vi "new8channelConvert.vi"(8 "Port 0":T1={"Port 0 Channel 0"=[0, 0, 0, 0, 0, 0, 0, 0, 0], "Port 0 Channel 1"=[0, 0, 0, 0, 0, 0, 0, 0, 0], "Port 0 Channel 2"=[0, 0, 0, 0, 0, 0, 0, 0, 0], "Port 0 Channel 3"=[0, 0, 0, 0, 0, 0, 0, 0, 0], "Port 0 Channel 4"=[0, 0, 0, 0, 0, 0, 0, 0, 0], "Port 0 Channel 5"=[0, 0, 0, 0, 0, 0, 0, 0, 0], "Port 0 Channel 6"=[0, 0, 0, 0, 0, 0, 0, 0, 0], "Port 0 Channel 7"=[0, 0, 0, 0, 0, 0, 0, 0, 0]}, 14 "采样率":i32=1, 18 "总时间（ms）":i32=10) -> (16 "单通道总采样点":i32, 19 "result":i32[](array[numeric]))   [LabVIEW 2021]
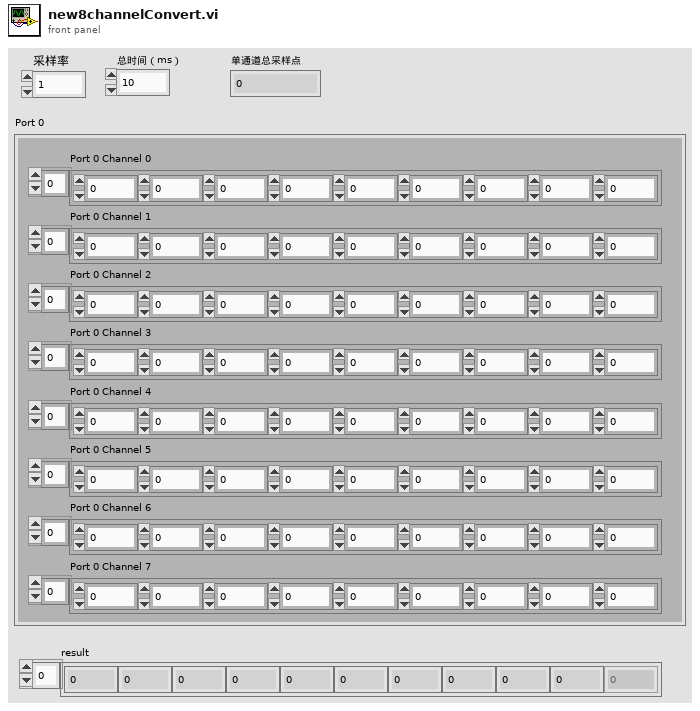
[diagram p1: front panel]
types:
  T1 = cluster{"Port 0 Channel 0":i32[], "Port 0 Channel 1":i32[], "Port 0 Channel 2":i32[], "Port 0 Channel 3":i32[], "Port 0 Channel 4":i32[], "Port 0 Channel 5":i32[], "Port 0 Channel 6":i32[], "Port 0 Channel 7":i32[]}
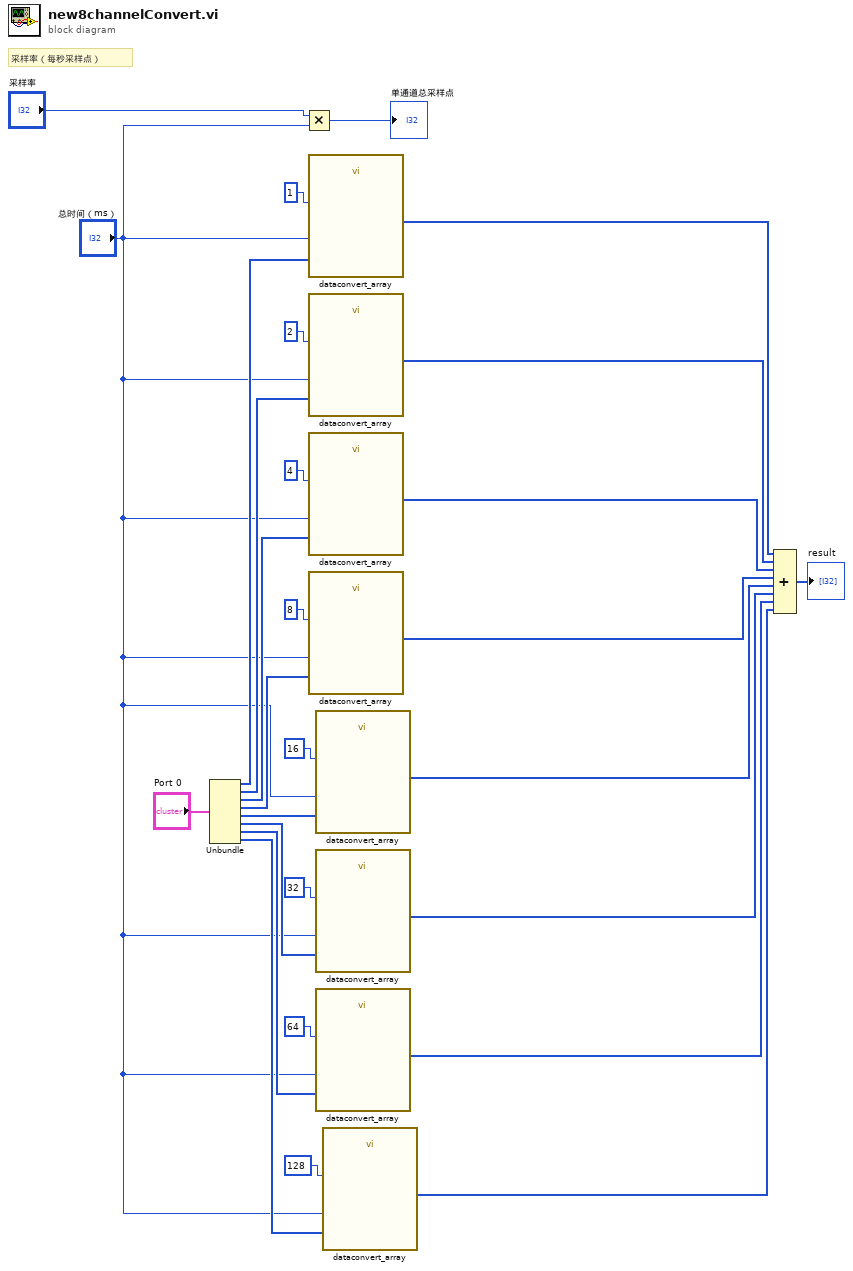
[diagram p0: block diagram]
diagram:
  # "采样率（每秒采样点）"
  n1 = Unbundle("Port 0") -> ("Port 0 Channel 0"=w20:i32[], "Port 0 Channel 1"=w19:i32[], "Port 0 Channel 2"=w18:i32[], "Port 0 Channel 3"=w17:i32[], "Port 0 Channel 4"=w16:i32[], "Port 0 Channel 5"=w15:i32[], "Port 0 Channel 6"=w14:i32[], "Port 0 Channel 7"=w13:i32[])
  n2 = Multiply(x="采样率", y="总时间（ms）") -> (x*y=→"单通道总采样点":i32)
  n3 = call "dataconvert_array.vi"("输入的TTL信号序列"=w20, "总时间（ms）"="总时间（ms）", "相乘倍数"=1) -> ("输出编码后的TTL序列"=w11:i32[])  [unwired: 8 in]
  n4 = call "dataconvert_array.vi"("输入的TTL信号序列"=w19, "总时间（ms）"="总时间（ms）", "相乘倍数"=2) -> ("输出编码后的TTL序列"=w10:i32[])  [unwired: 8 in]
  n5 = call "dataconvert_array.vi"("输入的TTL信号序列"=w18, "总时间（ms）"="总时间（ms）", "相乘倍数"=4) -> ("输出编码后的TTL序列"=w9:i32[])  [unwired: 8 in]
  n6 = call "dataconvert_array.vi"("输入的TTL信号序列"=w17, "总时间（ms）"="总时间（ms）", "相乘倍数"=8) -> ("输出编码后的TTL序列"=w8:i32[])  [unwired: 8 in]
  n7 = call "dataconvert_array.vi"("输入的TTL信号序列"=w16, "总时间（ms）"="总时间（ms）", "相乘倍数"=16) -> ("输出编码后的TTL序列"=w7:i32[])  [unwired: 8 in]
  n8 = call "dataconvert_array.vi"("输入的TTL信号序列"=w15, "总时间（ms）"="总时间（ms）", "相乘倍数"=32) -> ("输出编码后的TTL序列"=w6:i32[])  [unwired: 8 in]
  n9 = call "dataconvert_array.vi"("输入的TTL信号序列"=w14, "总时间（ms）"="总时间（ms）", "相乘倍数"=64) -> ("输出编码后的TTL序列"=w5:i32[])  [unwired: 8 in]
  n10 = call "dataconvert_array.vi"("输入的TTL信号序列"=w13, "总时间（ms）"="总时间（ms）", "相乘倍数"=128) -> ("输出编码后的TTL序列"=w4:i32[])  [unwired: 8 in]
  n11 = Compound Arithmetic op=ADD(w11, w10, w9, w8, w7, w6, w5, w4) -> (→"result":i32[])
